vi "initHandler.vi"(8 "error in (no error)":errorcluster, 9 "Name":string, 10 "Level":T1(ring), 11 "Handler in":refnum<class "Handler.lvclass">) -> (0 "error out":errorcluster, 3 "Handler out":refnum<class "Handler.lvclass">)   [LabVIEW 2017, in "Error Log.lvlib" / "Handler.lvclass"]
uses:
  Handler.lvclass
  Handler.lvclass/Handler.ctl
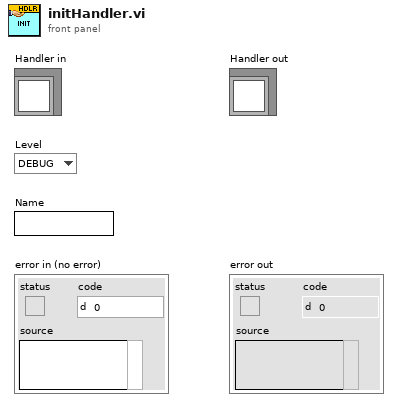
[diagram p1: front panel]
types:
  T1 = enum16{"DEBUG", "INFO", "WARNING", "ERROR", "CRITICAL"}
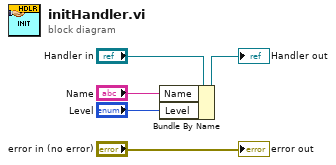
[diagram p0: block diagram]
diagram:
  n1 = Bundle By Name(cluster="Handler in", "Name"="Name", "Level"="Level") -> (→"Handler out":refnum<class "Handler.lvclass">)
  "error out" <- "error in (no error)"
